vi "CopyToTelemetryFIFO.vi"(11 "SourceFIFO":refnum<k21>="TelemetryFIFO") -> ()   [LabVIEW 2018]
uses:
  <vilib>/rvi/Emulation/niFpgaGetClockAttributes.vi
  <vilib>/rvi/Emulation/niFpgaSctlEmulationGetInTimedLoop.vi
  <vilib>/rvi/Emulation/niFpgaEmulationReportErrorSimple.vi
  <vilib>/rvi/DataTransferAndStorage/Container/Common/niFpgaContainerExecOnDevCompGetState.vi
  <vilib>/rvi/Emulation/niFpgaEmulationIsFPGAContextNoSignature.vi
  <vilib>/rvi/errors/niFpgaSetErrorForExecOnDevCompSimple.vi
  <vilib>/rvi/eio/common/nirviEmuReportErrorAndStop.vi
  <vilib>/rvi/DataTransferAndStorage/Container/Common/niFpgaContainerGetUniqueNameForEmu.vi
  <vilib>/rvi/FIFO/Fifo_Resource/nirvififoEmulationSetSize.vi
  <vilib>/rvi/FIFO/Fifo_Resource/nirviFifoEmulationQueueMgr.vi
  <instcachedir>/0/nirviFifoEmulationQueueMgr_E5CAEC123FF24DC58D834DCA3CDAA9B5.lvgen/nirviFifoEmulationQueueMgr_E5CAEC123FF24DC58D834DCA3CDAA9B5_022.vi
  <vilib>/rvi/FIFO/Fifo_Resource/nirvififoEmulationDetermineInputValidOut.vi
  <vilib>/rvi/FIFO/Fifo_Resource/nirvififoEmulationCreateLock.vi
  <vilib>/rvi/Emulation/niFpgaProcessEmulError.vi
  <vilib>/rvi/FIFO/Fifo_Resource/nirvififoEmulationObtainLock.vi
  <vilib>/rvi/FIFO/Fifo_Resource/nirvififoEmulationReleaseLock.vi
  <vilib>/rvi/occurrence/nirviWaitOnOccurrenceBase.vi
  <vilib>/rvi/errors/nirviReportUnexpectedCaseInternalError.vi
  <vilib>/rvi/errors/nirviReportUnexpectedCaseInternalError (U32).vi
  <vilib>/Utility/error.llb/Clear Errors.vi
  <vilib>/rvi/interface/RandomDataEmulation/niFpgaRandomDataHandleErrors.vi
  <vilib>/rvi/Emulation/niFpgaCriticalErrorInLSC.vi
  <vilib>/rvi/DataTransferAndStorage/Container/XNode/niFpgaContainer.xnode
  <vilib>/rvi/FIFO/Fifo_Resource/niFpgaFifoEmulationRefIn.vi
  <vilib>/rvi/FIFO/Fifo_Resource/nirvififoEmulationWrite.vi
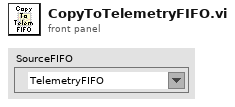
[diagram p1: front panel]
types:
  T1 = cluster{"DataType":enum8{"U8", "U16", "U32", "U64", "I8", "I16", "I32", "I64", "SGL"}, "Mode":enum8{"=", "+", "-", "|"}, "Field":enum16{"None", "AnalogInputSampleCount", "AnalogInputSampleTimestamp", "AnalogInputRaw1", "AnalogInputRaw2", "AnalogInputRaw3", "AnalogInputRaw4", "AnalogInputRaw5", "AnalogInputRaw6", "AnalogInputRaw7", "AnalogInputRaw8", "AnalogInputRaw9", "AnalogInputRaw10", "AnalogInputRaw11", "AnalogInputRaw12", "AnalogInputRaw13", "AnalogInputRaw14", "AnalogInputRaw15", "AnalogInputRaw16", "DigitalInputSampleCount", "DigitalInputSampleTimestamp", "DigitalInputStates", "ThermocoupleSampleCount", "ThermocoupleSampleTimestamp", "ThermocoupleRaw1", "ThermocoupleRaw2", "ThermocoupleRaw3", "ThermocoupleRaw4", "ThermocoupleRaw5", "ThermocoupleRaw6", "ThermocoupleRaw7", "ThermocoupleRaw8", "ThermocoupleRaw9", "ThermocoupleRaw10", "ThermocoupleRaw11", "ThermocoupleRaw12", "ThermocoupleRaw13", "ThermocoupleRaw14", "ThermocoupleRaw15", "ThermocoupleRaw16", "WindSensorTxBytes", "WindSensorTxFrames", "WindSensorRxBytes", "WindSensorRxFrames", "WindSensorErrorTimestamp", "WindSensorErrorCode", "WindSensorSampleTimestamp", "WindSensorXRaw", "WindSensorYRaw", "WindSensorZRaw", "WindSensorSonicTempRaw", "WindSensorDiagWord", "WindSensorRecordCount", "FlowSensorTxBytes", "FlowSensorTxFrames", "FlowSensorRxBytes", "FlowSensorRxFrames", "FlowSensorErrorTimestamp", "FlowSensorErrorCode", "FlowSensorSampleTimestamp", "FlowSensorSignalStrength", "FlowSensorFlowRate", "FlowSensorNetTotalizer", "FlowSensorPositiveTotalizer", "FlowSensorNegativeTotalizer", "FlowSensorTemperature1", "FlowSensorTemperature2", "VFDTxBytes", "VFDTxFrames", "VFDRxBytes", "VFDRxFrames", "VFDErrorTimestamp", "VFDErrorCode", "VFDSampleTimestamp", "VFDVelocityBits", "VFDDiagnosticCode", "VFDFrequencyCommand", "VFDOutputFrequency", "VFDOutputCurrent", "VFDDCBusVoltage", "VFDOutputVoltage"}, "Data":u64}
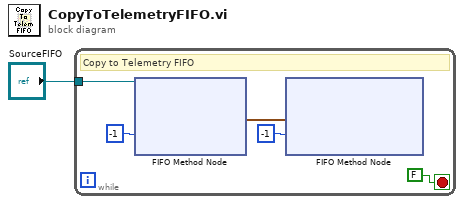
[diagram p0: block diagram]
diagram:
  n1 = while {
    tunnel: "SourceFIFO" -> [w6]
    stop <- FALSE stop-if-true
    # "Copy to Telemetry FIFO"
    n2 = xnode ("FIFO Method Node")("Timeout"=-1, "FIFO In"=w6) -> ("Element"=w5:T1)  [unwired: 2 out]
    n3 = xnode ("FIFO Method Node")("Element"=w5, "Timeout"=-1) -> ()  [unwired: 1 in, 2 out]
  }
